vi "Sleep.vi"(8 "error in (no error)":errorcluster, 11 "PCA in":refnum<class "PCA.lvclass">) -> (0 "error out":errorcluster, 3 "PCA out":refnum<class "PCA.lvclass">)   [LabVIEW 2022 SP3, in "PCA9685.lvlib" / "PCA.lvclass"]
uses:
  PCA.lvclass
  PCA.lvclass/PCA.ctl
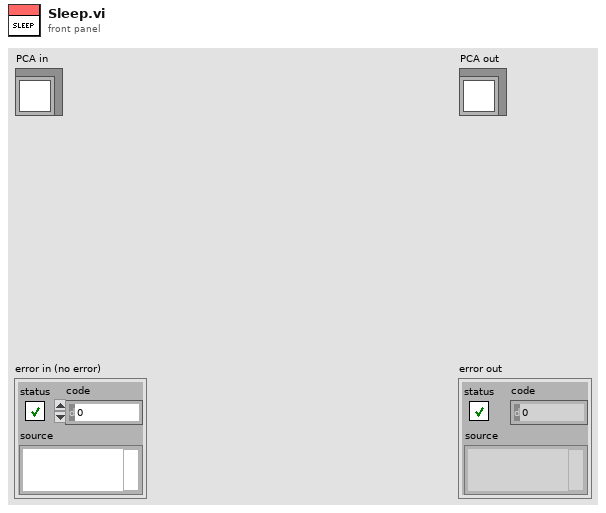
[diagram p1: front panel]
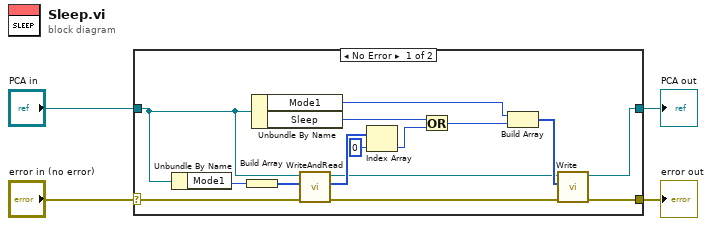
[diagram p0: block diagram]
diagram:
  n1 = case shown="No Error" "error in (no error)" {
    selector: "error in (no error)" -> [w19 w21]
    tunnel: [w10 w21] -> w3
    tunnel: [w5 w20] -> w1
    tunnel: "PCA in" -> [w16 w20]
    frame No Error {
      n2 = Unbundle By Name(w16) -> ("Mode1"=w18:u8)
      n3 = Build Array(w18) -> (w17:u8[])
      n4 = Unbundle By Name(w16) -> ("Mode1"=w8:u8, "Sleep"=w15:u8)
      n5 = call "WriteAndRead.vi"("error in (no error)"=w19, "Data"=w17, "PCA in"=w16) -> ("error out"=w11:errorcluster, "Data 2"=w13:u8[], "PCA out"=w6:refnum<class "PCA.lvclass">)  [unwired: 6 in]
      n6 = Index Array(array=w13, index=0) -> (element=w14:u8)
      n7 = Or(x=w15, y=w14) -> (x .or. y?=w9:u8)
      n8 = Build Array(w8, w9) -> (w7:u8[])
      n9 = call "Write.vi"("error in (no error)"=w11, "Data"=w7, "PCA in"=w6) -> ("error out"=w10:errorcluster, "PCA out"=w5:refnum<class "PCA.lvclass">)  [unwired: 7 in]
    }
    frame Error {
    }
  }
  "error out" <- w3
  "PCA out" <- w1
